vi "test Set ObjectType_3.vi"(11 "Test Entry":refnum<class "Test Object Entry.lvclass">) -> (0 "error out":errorcluster, 3 "Test Entry":refnum<class "Test Object Entry.lvclass">)   [LabVIEW 2020, in "Test Object Entry.lvclass"]
uses:
  Test Object Entry.lvclass
  C:/Program Files/National Instruments/LabVIEW 2026/vi.lib/Astemes/LUnit/Test Case.lvclass
  source/Object Entry/Object Entry.lvclass
  source/Object Entry/Object Entry.lvclass/Object Entry.ctl
  <vilib>/Astemes/LUnit/Test Case.lvclass/Test Case.ctl
  source/Typedefs/Object Type.ctl
  aa63150e-3d96-4f0c-8081-450150bc22f9.vi
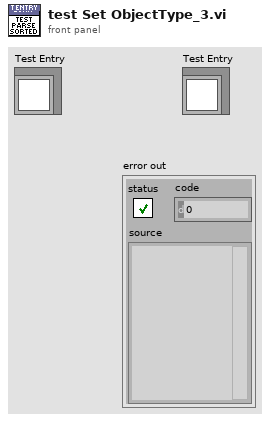
[diagram p1: front panel]
types:
  T1 = typedef "Object Type.ctl" = u8
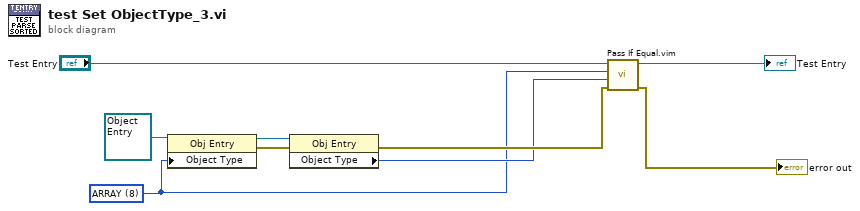
[diagram p0: block diagram]
diagram:
  w1 = T1 8 items=["NULL"=0, "DOMAIN"=2, "DEFTYPE"=5, "DEFSTRUCT"=6, "VAR"=7, "ARRAY"=8, "RECORD"=9] ("Object Type")
  n1 = property class="Obj Entry"(reference=refnum<class "Object Entry.lvclass"> refnum ("CANopen.lvlib:Obj Entry"), "Object Type"=w1) -> (reference out=w4:refnum<class "Object Entry.lvclass">, error out=w6:errorcluster)  [unwired: 1 in]
  n2 = property class="Obj Entry"(reference=w4, error in=w6) -> (error out=w5:errorcluster, "Object Type"=w2:T1)  [unwired: 1 out]
  n3 = call "Pass If Equal.vim"("error in (no error)"=w5, "Actual"=w2, "Expected"=w1, "LUnit Test Case In"="Test Entry") -> ("error out"=→"error out":errorcluster, "LUnit Test Case Out"=→"Test Entry":refnum<class "Test Object Entry.lvclass">)  [unwired: 6 in]
